vi "ex_WriteDataTDMS.vi"(0 "file path":path, 1 "first call":bool, 2 "Lock file":bool=TRUE, 3 "Signals":waveform(dbl)[](array[waveform]), 4 "overwrite_mode_multi":T8(ring)=enum."overwrite & backup", 5 "overwrite_mode":T9(ring)=enum."overwrite & backup", 7 "error in (no error)":errorcluster, 8 "file dialog?":bool, 9 "Description":string, 12 "multi_file":bool, 13 "Comment":string, 14 "new file?":bool, 15 "Simulate Non-First Call":bool, 16 "file params":T6={"delimiter"="\t", "origin time"=timestamp(0 s since 1904-01-01), "Flags"={"include col headings?"=TRUE, "x_columns"=0, "col headings always?"=TRUE, "time preference"=0, "hide col headings"=FALSE}, "Decimal Separator"=""} {"Flags"."time preference" items=["Absolute", "Relative"]; "Flags"."x_columns" items=["None", "One", "Multiple"]; "origin time" format="%<%X\n%x>T"}, 23 "append info in":T5, 25 "DAQmx Task":T1) -> (17 "operator cancelled?":bool, 20 "file path out":path, 21 "bytes written":i32, 24 "append info out":T5, 27 "error out":errorcluster)   [LabVIEW 2017]
uses:
  <vilib>/express/express output/ExFileWriteBlock.llb/ex_WriteFileParams.ctl
  <vilib>/express/express input/ExFileReadBlock.llb/ex_ReadFileParams.ctl
  <vilib>/Platform/express/TDMExpress.llb/ex_appendInfoTDM.ctl
  <vilib>/express/express shared/ex_EditUserDefinedProperties/ex_userdefproperties.ctl
  <vilib>/express/express shared/ExFile.llb/ex_userDefProperty.ctl
  <vilib>/express/express shared/ex_EditUserDefinedProperties/usiDataType.ctl
  <vilib>/express/express shared/ExFile.llb/ex_propertySource.ctl
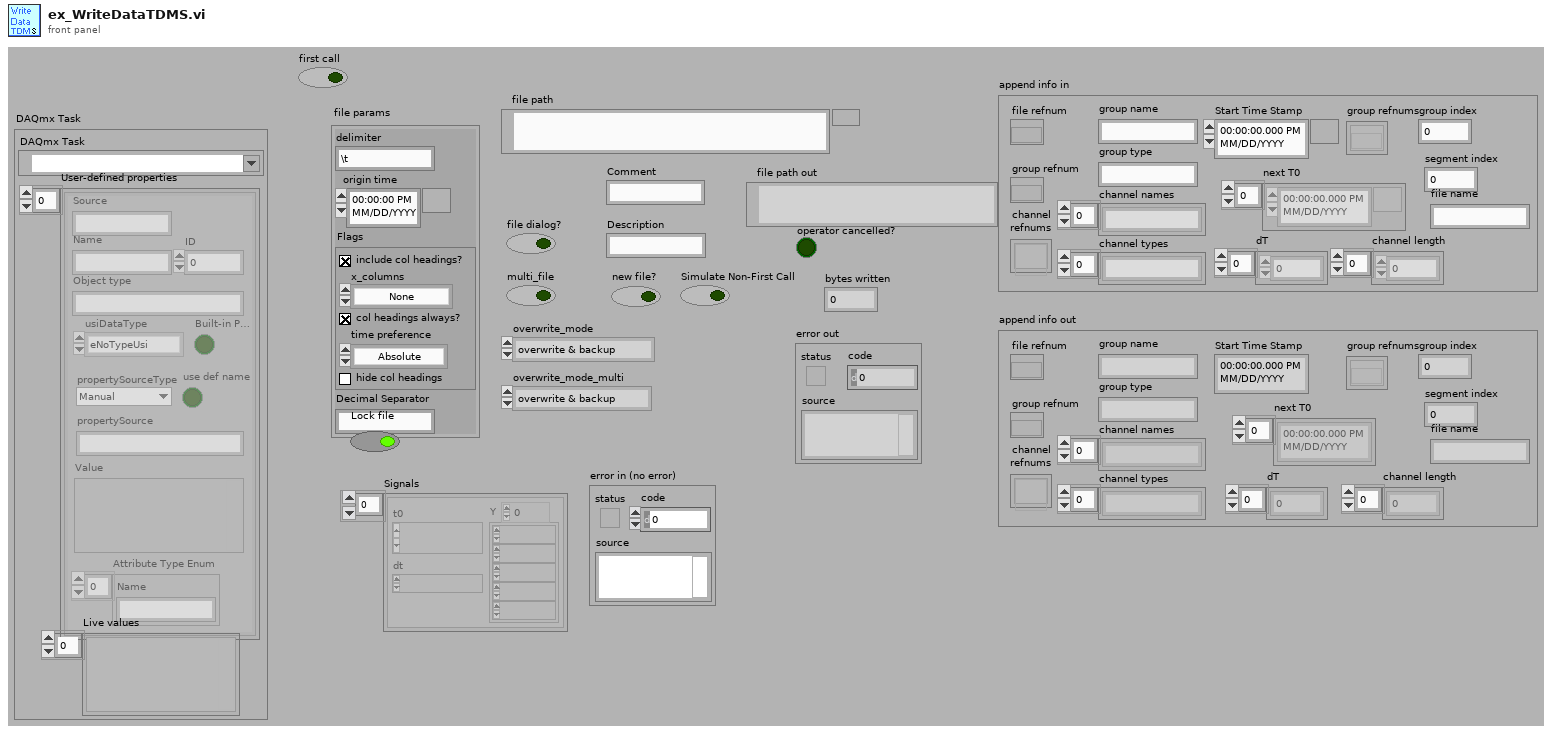
[diagram p1: front panel]
types:
  T1 = typedef "ex_userdefproperties.ctl" = cluster{"DAQmx Task":refnum<k21>, "User-defined properties":T2[], "Live values":variant[]}
  T2 = typedef "ex_userDefProperty.ctl" = cluster{"Name":string, "Object type":string, "usiDataType":T3, "propertySourceType":T4, "propertySource":string, "Value":variant, "ID":i32, "use def name":bool, "Source":string, "Built-in Prop":bool, "Attribute Type Enum":string[]}
  T3 = typedef "usiDataType.ctl" = enum16{"eNoTypeUsi", "eInt8Usi", "eInt16Usi", "eInt32Usi", "eInt64Usi", "eUInt8Usi", "eUInt16Usi", "eUInt32Usi", "eUInt64Usi", "eFloat32Usi", "eFloat64Usi", "- 0", "- 1", "- 2", "- 3", "- 4", "- 5", "- 6", "- 7", "- 8", "- 9", "eString8Usi", "eString16Usi", "eStringUsi", "eEnumUsi", "- 10", "- 11", "- 12", "- 13", "- 14", "eTimeUsi", "- 15", "- 16", "- 17", "- 18", "- 19", "- 20", "- 21", "- 22", "- 23", "eInstanceUsi", "eStoreUsi"}
  T4 = typedef "ex_propertySource.ctl" = enum16{"Manual", "System", "DAQmx Channel", "Terminal", "Ignore"}
  T5 = typedef "ex_appendInfoTDM.ctl" = cluster{"channel\nrefnums":refnum<k20>[], "channel names":string[], "channel types":string[], "file refnum":refnum<k20>, "group refnum":refnum<k20>, "group name":string, "group type":string, "next T0":timestamp[], "dT":dbl[], "Start Time Stamp":timestamp, "channel length":u32[], "group index":u32, "group refnums":refnum<k20>[], "file name":string, "segment index":u32}
  T6 = typedef "ex_WriteFileParams.ctl" = cluster{"delimiter":string, "origin time":timestamp, "Flags":T7, "Decimal Separator":string}
  T7 = typedef "ex_ReadFileParams.ctl" = cluster{"include col headings?":bool, "x_columns":u16, "col headings always?":bool, "time preference":u16, "hide col headings":bool}
  T8 = enum16{"overwrite", "overwrite & backup", "next avail"}
  T9 = enum16{"overwrite", "overwrite & backup", "append", "next avail"}
  T10 = cluster{"Start Timestamp":timestamp, "Timestamp":timestamp, "Relative Time?":bool, "X Dimension":string, "Signal Name":string, "Y Units":string, "X0":timestamp, "dX":dbl, "nPoints":i32}[]
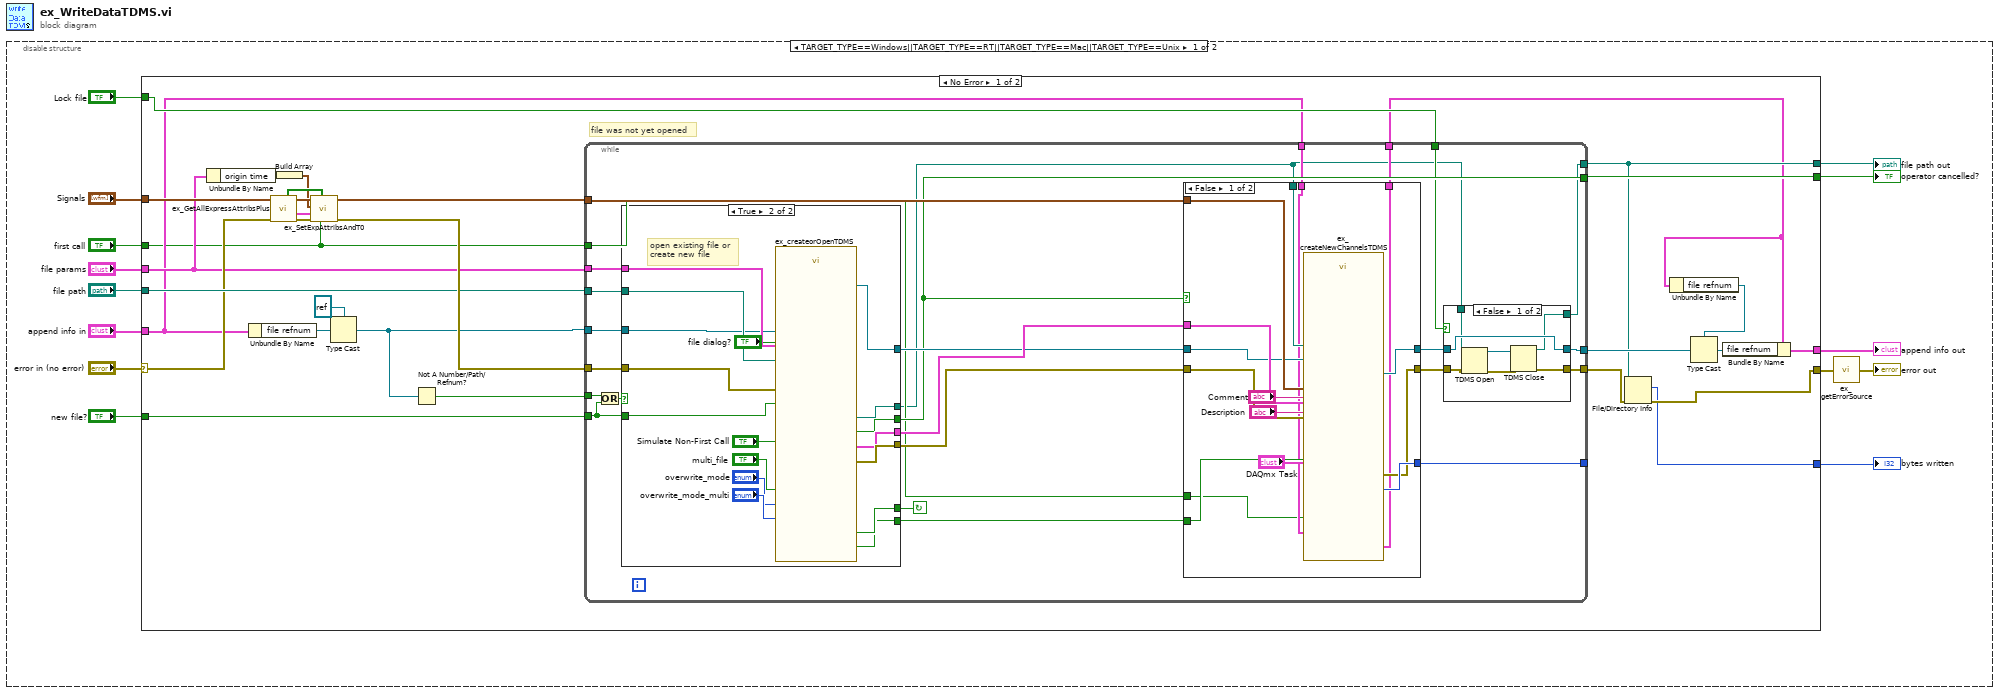
[diagram p0: block diagram]
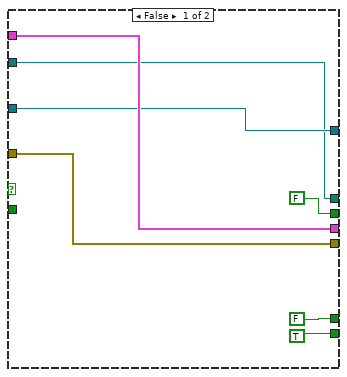
[diagram p2: hidden frame]
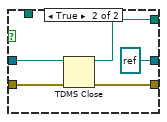
[diagram p3: hidden frame]
diagram:
  n1 = disable-structure shown="TARGET_TYPE==Windows||TARGET_TYPE==RT||TARGET_TYPE==Mac||TARGET_TYPE==Unix" {
    frame condition #0 (active) {
      n2 = case shown="No Error" "error in (no error)" {
        selector: "error in (no error)" -> [w32 w126]
        tunnel: [w19 w126] -> w14
        tunnel: "Signals" -> [w34 _]
        tunnel: "new file?" -> [w41 _]
        tunnel: "file params" -> [w26 _]
        tunnel: [w25 w125] -> w7
        tunnel: "file path" -> [w43 w124]
        tunnel: "append info in" -> [w22 w125]
        tunnel: "Lock file" -> [w42 _]
        tunnel: [w18 w124] -> w6
        tunnel: [w39 _] -> w5
        tunnel: [w17 _] -> w4
        tunnel: "first call" -> [w21 _]
        frame No Error {
          # "file was not yet opened"
          n3 = Unbundle By Name(w26) -> ("origin time"=w31:timestamp)
          n4 = Unbundle By Name(w22) -> ("file refnum"=w29:refnum<k20>)
          n5 = call <vilib>:"ex_GetAllExpressAttribsPlus.vi"("error in"=w32, "Signals in"=w34) -> ("error out"=w38:errorcluster, "All Express Wave Attributes Plus"=w37:T10, "Signals out"=w36:waveform(dbl)[], "Time Attribs Not Found"=w35:bool[])  [unwired: 6 out]
          n6 = Build Array(w31) -> (w30:timestamp[])
          n7 = call <vilib>:"ex_SetExpAttribsAndT0.vi"("Latch Origin TS? (T)"=w21, "Set? (T if empty)"=w35, "error in (no error)"=w38, "Express Attributes Plus in"=w37, "Origin Timestamps"=w30, "Signals"=w36) -> ("error out"=w44:errorcluster, "Signals With Attributes"=w33:waveform(dbl)[])  [unwired: 4 out]
          n8 = Type Cast(type=refnum<k34> refnum ("tdms file out"), x=w29) -> (*(type *) &x=w27:refnum<k34>)
          n9 = Not A Number/Path/Refnum?(number/path/refnum=w27) -> (NaN/Path/Refnum?=w40:bool)
          n10 = while {
            tunnel: w44 -> [w69]
            tunnel: w41 -> [w55]
            tunnel: w43 -> [w68]
            tunnel: [w46] -> w18
            tunnel: [w51] -> w39
            tunnel: [w64] -> w20
            tunnel: [w67] -> _
            tunnel: w26 -> [w66]
            tunnel: [w63] -> w24
            tunnel: w42 -> [w47]
            tunnel: w27 -> [w59]
            tunnel: w33 -> [w60]
            tunnel: w40 -> [w56]
            tunnel: w22 -> [w50]
            tunnel: [w49] -> w16
            tunnel: w21 -> [w48]
            stop <- w65 continue-if-true
            n11 = Or(x=w56, y=w55) -> (x .or. y?=w57:bool)
            n12 = case shown="True" w57 {
              tunnel: w69 -> [w74 w93]
              tunnel: w68 -> [w73 w92]
              tunnel: w66 -> [w76 w90]
              tunnel: [FALSE ("keep loop going") w85] -> w65
              tunnel: [w73 w84] -> w45
              tunnel: [w74 w83] -> w62
              tunnel: [w76 w82] -> w61
              tunnel: w55 -> [_ w81]
              tunnel: w59 -> [w75 w80]
              tunnel: [w75 w79] -> w58
              tunnel: [FALSE ("dialog was cancelled") w78] -> w51
              tunnel: [TRUE ("keep loop going") w77] -> w54
              frame False {
              }
              frame True {
                # "open existing file or\ncreate new file"
                n13 = call <vilib>:"ex_createorOpenTDMS.vi"("file path in"=w92, "overwrite_mode_multi"="overwrite_mode_multi", "overwrite_mode"="overwrite_mode", "tdms file in"=w80, "file dialog?"="file dialog?", "error in (no error)"=w93, "file params"=w90, "multi_file"="multi_file", "new file?"=w81, "Simulate Non-First Call"="Simulate Non-First Call") -> ("new file was created"=w77:bool, "file path out"=w84:path, "dialog was cancelled"=w78:bool, "keep loop going"=w85:bool, "tdms file out"=w79:refnum<k34>, "file params out"=w82:T6, "error out"=w83:errorcluster)  [unwired: 3 out]
              }
            }
            n14 = case shown="False" w51 {
              tunnel: w61 -> [w116 _]
              tunnel: [w118 w123] -> w52
              tunnel: w62 -> [w120 w123]
              tunnel: [w119 _] -> w67
              tunnel: [w117 w122] -> w53
              tunnel: w58 -> [w109 w122]
              tunnel: w60 -> [w115 _]
              tunnel: w54 -> [w114 _]
              tunnel: w45 -> [w110 _]
              tunnel: w50 -> [w108 w121]
              tunnel: [w107 w121] -> w49
              tunnel: w48 -> [w106 _]
              frame False {
                n15 = call <vilib>:"ex_createNewChannelsTDMS.vi"("DAQmx Task"="DAQmx Task", "tdms file in"=w109, "append info in"=w108, "signals"=w115, "file params"=w116, "File path"=w110, "is first call"=w106, "error in (no error)"=w120, "Comment"="Comment", "Description"="Description", "write file properties"=w114) -> ("append info out"=w107:T5, "tdms file out"=w117:refnum<k34>, "bytes written"=w119:i32, "error out"=w118:errorcluster)  [unwired: 1 out]
              }
              frame True {
              }
            }
            n16 = case shown="False" w47 {
              tunnel: w52 -> [w99 w105]
              tunnel: [w97 w103] -> w64
              tunnel: w53 -> [w100 w104]
              tunnel: [w100 refnum<k34> refnum ("tdms file out")] -> w63
              tunnel: [w95 w101] -> w46
              tunnel: w45 -> [w94 _]
              frame False {
                n17 = TDMS Open(8:w99, 11:w94) -> (0:w98:errorcluster, 3:w96:refnum<k34>)  [unwired: 5 in]
                n18 = TDMS Close(8:w98, 11:w96) -> (0:w97:errorcluster, 3:w95:path)
              }
              frame True {
                n19 = TDMS Close(8:w105, 11:w104) -> (0:w103:errorcluster, 3:w101:path)
              }
            }
          }
          n20 = File/Directory Info(path=w18, error in=w20) -> (size=w17:i64, error out=w19:errorcluster)  [unwired: 5 out]
          n21 = Unbundle By Name(w16) -> ("file refnum"=w15:refnum<k20>)
          n22 = Type Cast(type=w15, x=w24) -> (*(type *) &x=w23:refnum<k20>)
          n23 = Bundle By Name(cluster=w16, "file refnum"=w23) -> (w25:T5)
        }
        frame Error {
        }
      }
      "append info out" <- w7
      "operator cancelled?" <- w5
      "file path out" <- w6
      "bytes written" <- w4
      n24 = call <vilib>:"ex_getErrorSource.vi"("error in (no error)"=w14) -> ("error out"=→"error out":errorcluster)
    }
    frame condition #1 {
    }
  }
